vi "SWERVE_SIM_READ_GYRO.vi"(9 "FPGA_Time_Seconds":dbl, 10 "vOmega":dbl, 11 "GyroDevRef":T1 {"Sample Rate" min=0.25 max=100.0 step=0.25}) -> (1 "Gyro_Cont_Deg":dbl)   [LabVIEW 2019]
uses:
  <vilib>/Rock Robotics/WPI/Gyro/WPI_GyroDevRef.ctl
  <vilib>/Rock Robotics/SystemInterfaces/AI/FPGA_AIChannel.ctl
  <vilib>/Rock Robotics/SystemInterfaces/spilib/spi_bus.ctl
  <vilib>/Rock Robotics/WPI/ThirdParty/JAS_Junk/TrajLib/Trajectory_Library.lvlib
panel:
  # "Analog"
  # "XRS"
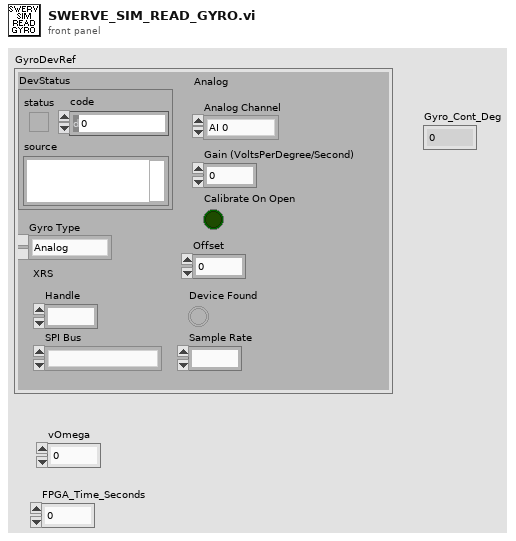
[diagram p1: front panel]
types:
  T1 = typedef "WPI_GyroDevRef.ctl" = cluster{"DevStatus":errorcluster, "Analog Channel":T2, "Gain (VoltsPerDegree/Second)":dbl, "Gyro Type":enum16{"Analog", "XRS450"}, "Handle":i32, "SPI Bus":T3, "Device Found":bool, "Sample Rate":dbl, "Calibrate On Open":bool, "Offset":dbl}
  T2 = typedef "FPGA_AIChannel.ctl" = enum8{"AI 0", "AI 1", "AI 2", "AI 3", "AI MXP 0", "AI MXP 1", "AI MXP 2", "AI MXP 3", "Invalid"}
  T3 = typedef "spi_bus.ctl" = enum16{"SPI On-Board, CS0", "SPI On-Board, CS1", "SPI On-Board, CS2", "SPI On-Board, CS3", "SPI MXP", "Invalid"}
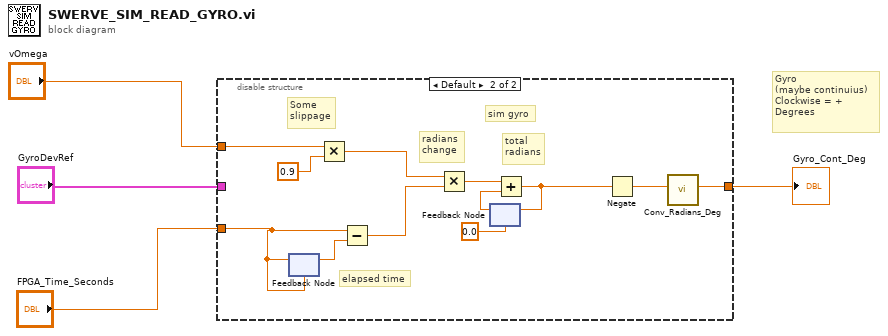
[diagram p0: block diagram]
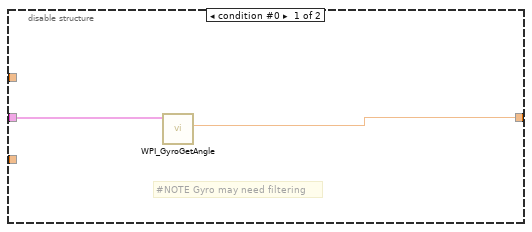
[diagram p2: hidden frame]
diagram:
  # "Gyro\n(maybe continuius)\nClockwise = +\nDegrees"
  n1 = disable-structure shown="Default" {
    disable-tunnel: "GyroDevRef" -> [w6 _]
    disable-tunnel: "vOmega" -> [_ w9]
    disable-tunnel: "FPGA_Time_Seconds" -> [_ w14]
    disable-tunnel: [w5 w12] -> w1
    frame condition #0 {
      # "#NOTE Gyro may need filtering"
      n2 = call <vilib>:"WPI_GyroGetAngle.vi"("GyroDevRef"=w6) -> ("Angle"=w5:dbl)  [unwired: 6 in, 4 out]
    }
    frame condition #1 (active) {
      # "Some \nslippage"
      # "elapsed time"
      # "total \nradians"
      # "radians \nchange"
      # "sim gyro"
      n3 = feedback #1(w14) -> (w15:dbl)
      n4 = feedback-in #1(w14) -> ()
      n5 = Multiply(x=w9, y=0.9) -> (x*y=w8:dbl)
      n6 = Subtract(x=w14, y=w15) -> (x-y=w13:dbl)
      n7 = Multiply(x=w8, y=w13) -> (x*y=w16:dbl)
      n8 = feedback #2(0.0) -> (w17:dbl)
      n9 = Add(x=w16, y=w17) -> (x+y=w11:dbl)
      n10 = feedback-in #2(w11) -> ()
      n11 = Negate(x=w11) -> (-x=w10:dbl)
      n12 = call <vilib>:"Conv_Radians_Deg.vi"("Radians"=w10) -> ("Degrees"=w12:dbl)  [unwired: 10 in]
    }
  }
  "Gyro_Cont_Deg" <- w1
